vi "HEALTH_LABVIEW_V4.vi"() -> ()   [LabVIEW 2026]
uses:
  <vilib>/addons/control/pid/NI_PID_pid.lvlib
  <vilib>/addons/control/pid/pid.llb/PID (DBL).vi
panel:
  out "INTERMEDIATE BLOCK LOWER RTD":dbl format="%.2f"
  out "INTERMEDIATE BLOCK LOWER RTD":dbl(graph)
  out "OUTLET TEMP (C)":dbl
  out "INLET TEMP (C)":dbl
  out "INLET PRESSURE (PSI)":dbl format="%.2f"
  out "INLET PRESSURE (PSI)":dbl(graph)
  out "PRESSURE DROP (PSI)":dbl format="%.2f"
  out "PRESSURE DROP (PSI)":dbl(graph)
  out "DELTA T (C)":dbl
  in  "ZEROING DELTA T OFFSET":dbl
  out "DELTA T (C)":dbl(graph)
  out "COOLANT FLOW (LPM)":dbl(graph)
  out "COOLANT FLOW (LPM)":dbl
  in  "HTR PROP GAIN":dbl=3.0
  in  "PUMP SPEED CONTROL VOLTAGE":dbl(knob) scale=0.0..5.0
  in  "PUMP ON/OFF":bool
  out "HX TEMPERATURE (C)":dbl(graph)
  out "HEATER POWER OUTPUT":dbl(knob) scale=0.0..100.0
  in  "TARGET HX TEMP (C)":dbl
  in  "HEATER ON/OFF":bool
  out "HX TEMP (C)":dbl format="%.2f"
  in  "stop":bool
  out "Error String":string
  out "error out":errorcluster
  out "ConnectionType Out":i32
  out "DeviceType Out":i32
  in  "Identifier":string="LJM_idANY"
  in  "ConnectionType":string="LJM_ctANY"
  in  "DeviceType":string="LJM_dtANY"
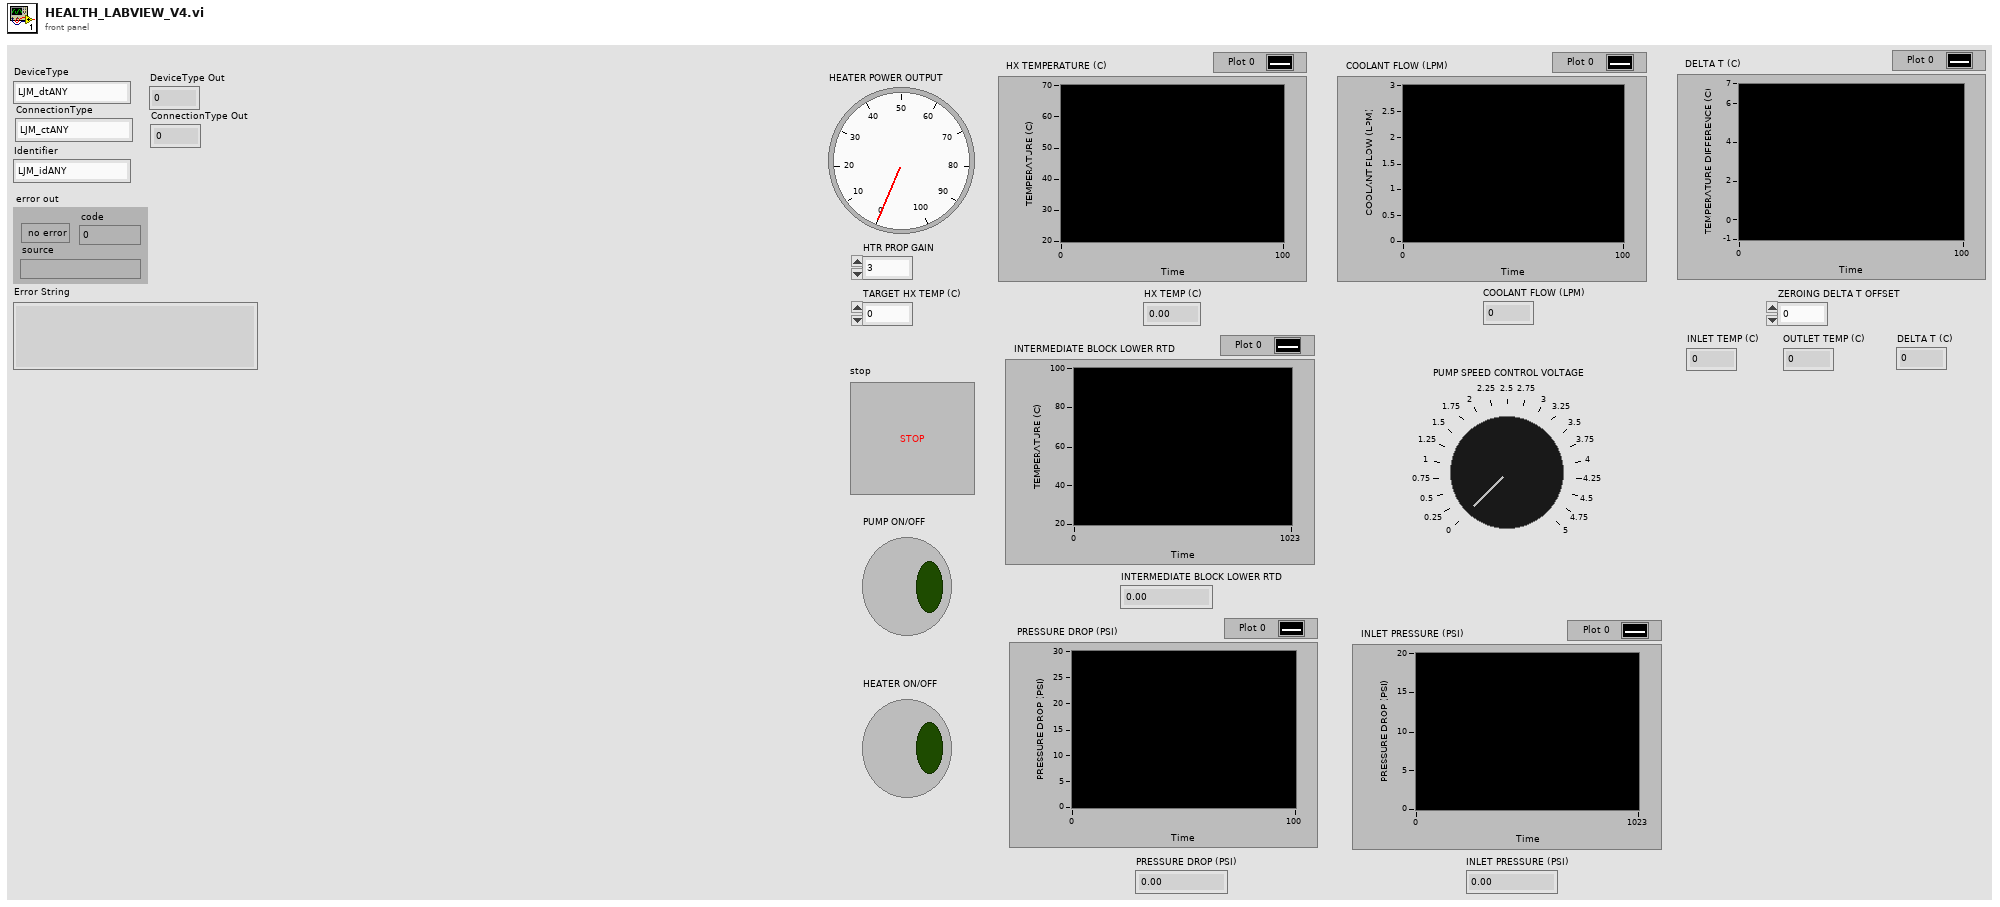
[diagram p1: front panel]
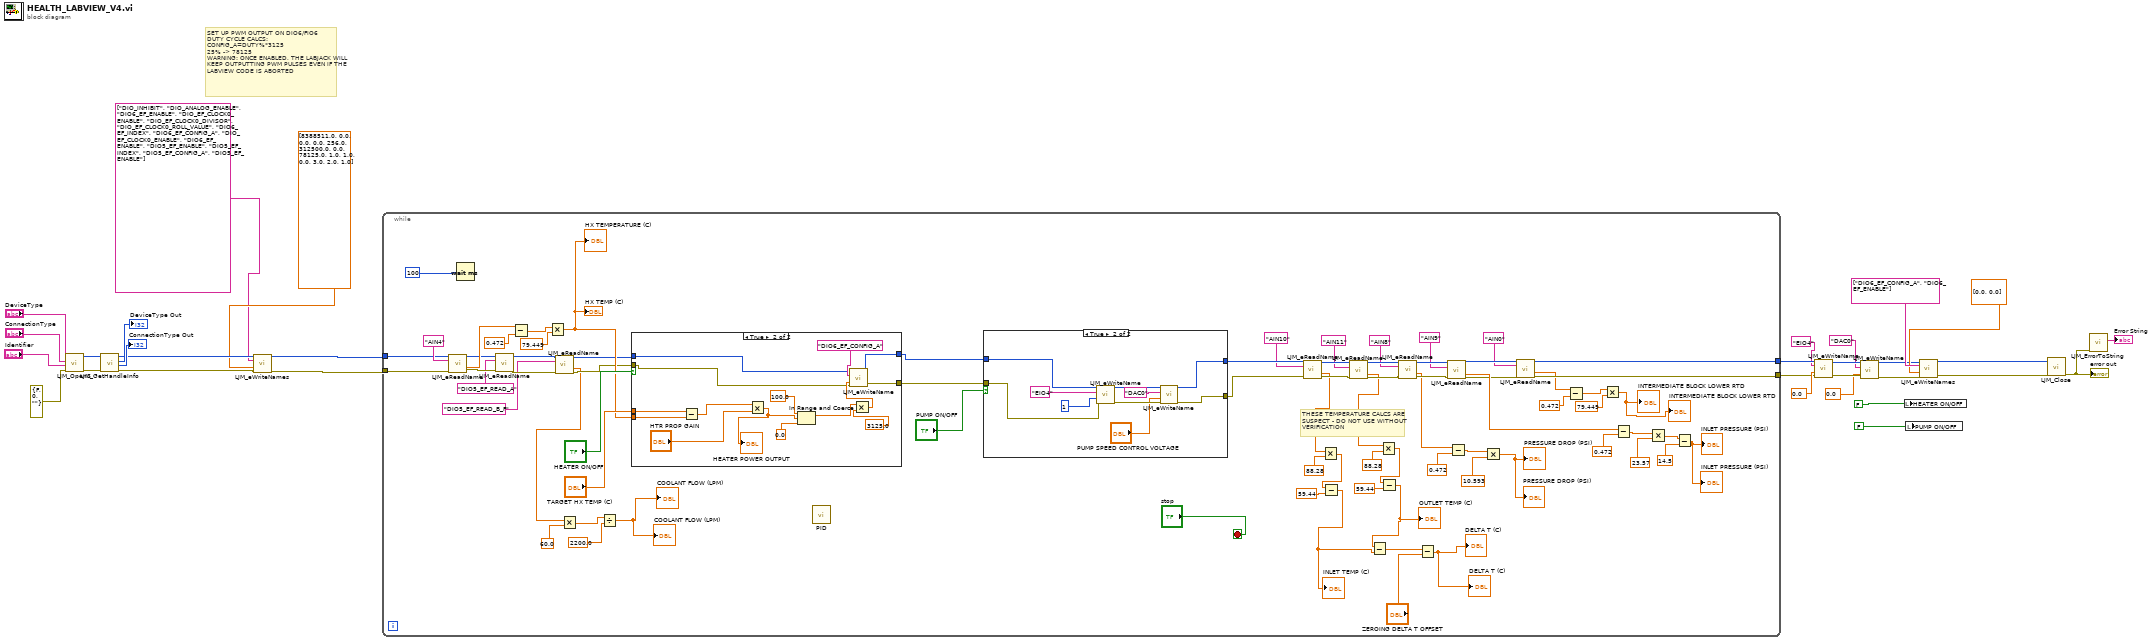
[diagram p0: block diagram]
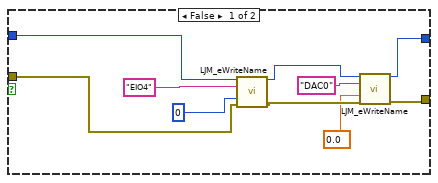
[diagram p2: hidden frame]
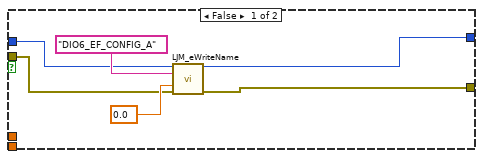
[diagram p3: hidden frame]
diagram:
  # "SET UP PWM OUTPUT ON DIO6/FIO6\nDUTY CYCLE CALCS:\nCONFIG_A=DUTY%*3125\n25% -> 78125\nWARNING: ONCE ENABLED, THE LABJACK WILL KEEP OUTPUTTING PWM PULSES EVEN IF THE LABVIEW CODE IS ABORTED"
  n1 = call "LJM_OpenS.vi"("error in"=errorcluster {"status"=FALSE, "code"=0, "source"=""} ("error in (no error)"), "Identifier"="Identifier", "ConnectionType"="ConnectionType", "DeviceType"="DeviceType") -> ("error out"=w31:errorcluster, "Handle"=w30:i32)  [unwired: 6 in]
  n2 = call "LJM_GetHandleInfo.vi"("error in"=w31, "Handle In"=w30) -> ("error out"=w21:errorcluster, "ConnectionType"=→"ConnectionType Out":i32, "DeviceType"=→"DeviceType Out":i32, "Handle Out"=w22:i32)  [unwired: 2 in, 4 out]
  n3 = call "LJM_eWriteNames.vi"("Handle In"=w22, "aNames"=string[] ["DIO_INHIBIT", "DIO_ANALOG_ENABLE", "DIO6_EF_ENABLE", "DIO_EF_CLOCK0_ENABLE", "DIO_EF_CLOCK0_DIVISOR", "DIO_EF_CLOCK0_ROLL_VALUE", "DIO6_EF_INDEX", "DIO6_EF_CONFIG_A", "DIO_EF_CLOCK0_ENABLE", "DIO6_EF_ENABLE", "DIO5_EF_ENABLE", "DIO5_EF_INDEX", "DIO5_EF_CONFIG_A", "DIO5_EF_ENABLE"], "aValuesIn"=dbl[] [8388511.0, 0.0, 0.0, 0.0, 256.0, 312500.0, 0.0, 78125.0, 1.0, 1.0, 0.0, 3.0, 2.0, 1.0], "error in"=w21) -> ("Handle Out"=w2:i32, "error out"=w1:errorcluster)  [unwired: 9 in, 1 out]
  n4 = while {
    tunnel: [w39] -> w9
    tunnel: w2 -> [w94]
    tunnel: w1 -> [w93]
    tunnel: [w40] -> w3
    stop <- "stop" stop-if-true
    # "THESE TEMPERATURE CALCS ARE SUSPECT - DO NOT USE WITHOUT VERIFICATION"
    n5 = call "LJM_eReadName.vi"("Handle In"=w94, "Name"="AIN4", "error in"=w93) -> ("Handle Out"=w92:i32, "Value"=w103:dbl, "error out"=w91:errorcluster)  [unwired: 10 in]
    n6 = Wait (ms)(milliseconds to wait=u32 100) -> ()  [unwired: 1 out]
    n7 = call "LJM_eReadName.vi"("Handle In"=w92, "Name"="DIO5_EF_READ_A", "error in"=w91) -> ("Handle Out"=w89:i32, "error out"=w86:errorcluster)  [unwired: 10 in, 1 out]
    n8 = Subtract(x=w103, y=0.472 ("Address 2")) -> (x-y=w106:dbl)
    n9 = Multiply(x=w106, y=79.449 ("Address 2")) -> (x*y=w98:dbl)
    "HX TEMP (C)" <- w98
    "HX TEMPERATURE (C)" <- w98
    n10 = call "LJM_eReadName.vi"("Handle In"=w89, "Name"="DIO5_EF_READ_B_F" ("DIO5_EF_READ_B_F"), "error in"=w86) -> ("Handle Out"=w88:i32, "Value"=w84:dbl, "error out"=w87:errorcluster)  [unwired: 10 in]
    n11 = Multiply(x=w84, y=60.0) -> (x*y=w82:dbl)
    n12 = Divide(x=w82, y=2200.0) -> (x/y=→"COOLANT FLOW (LPM)" →"COOLANT FLOW (LPM)":dbl)
    n13 = case shown="True" "HEATER ON/OFF" {
      tunnel: [w132 w148] -> w95
      tunnel: [w133 w147] -> w96
      tunnel: "TARGET HX TEMP (C)" -> [_ w143]
      tunnel: w98 -> [_ w142]
      tunnel: w88 -> [w129 w139]
      tunnel: w87 -> [w128 w138]
      frame False {
        n14 = call "LJM_eWriteName.vi"("Handle In"=w129, "Name"="DIO6_EF_CONFIG_A", "Value"=0.0, "error in"=w128) -> ("Handle Out"=w133:i32, "error out"=w132:errorcluster)  [unwired: 10 in]
      }
      frame True {
        n15 = Subtract(x=w143, y=w142) -> (x-y=w140:dbl)
        n16 = Multiply(x=w140, y="HTR PROP GAIN") -> (x*y=w137:dbl)
        "HEATER POWER OUTPUT" <- w137
        n17 = In Range and Coerce(upper limit=100.0, x=w137, lower limit=0.0) -> (coerced(x)=w134:dbl)  [unwired: 1 out]
        n18 = Multiply(x=w134, y=3125.0) -> (x*y=w145:dbl)
        n19 = call "LJM_eWriteName.vi"("Handle In"=w139, "Name"="DIO6_EF_CONFIG_A", "Value"=w145, "error in"=w138) -> ("Handle Out"=w147:i32, "error out"=w148:errorcluster)  [unwired: 10 in]
      }
    }
    n20 = call-poly <vilib>:"PID.vi"() -> ()  [unwired: 10 in, 2 out]
    n21 = case shown="True" "PUMP ON/OFF" {
      tunnel: w96 -> [w115 w125]
      tunnel: w95 -> [w114 w124]
      tunnel: [w110 w119] -> w75
      tunnel: [w109 w120] -> w79
      frame False {
        n22 = call "LJM_eWriteName.vi"("Handle In"=w115, "Name"="EIO4", "Value"=0, "error in"=w114) -> ("Handle Out"=w112:i32, "error out"=w111:errorcluster)  [unwired: 10 in]
        n23 = call "LJM_eWriteName.vi"("Handle In"=w112, "Name"="DAC0", "Value"=0.0, "error in"=w111) -> ("Handle Out"=w109:i32, "error out"=w110:errorcluster)  [unwired: 10 in]
      }
      frame True {
        n24 = call "LJM_eWriteName.vi"("Handle In"=w125, "Name"="EIO4", "Value"=1, "error in"=w124) -> ("Handle Out"=w121:i32, "error out"=w122:errorcluster)  [unwired: 10 in]
        n25 = call "LJM_eWriteName.vi"("Handle In"=w121, "Name"="DAC0", "Value"="PUMP SPEED CONTROL VOLTAGE", "error in"=w122) -> ("Handle Out"=w120:i32, "error out"=w119:errorcluster)  [unwired: 10 in]
      }
    }
    n26 = call "LJM_eReadName.vi"("Handle In"=w79, "Name"="AIN10", "error in"=w75) -> ("Handle Out"=w78:i32, "Value"=w67:dbl, "error out"=w74:errorcluster)  [unwired: 10 in]
    n27 = Multiply(x=w67, y=88.28) -> (x*y=w65:dbl)
    n28 = Subtract(x=w65, y=59.44) -> (x-y=w45:dbl)
    "INLET TEMP (C)" <- w45
    n29 = call "LJM_eReadName.vi"("Handle In"=w78, "Name"="AIN11" ("Name 2"), "error in"=w74) -> ("Handle Out"=w77:i32, "Value"=w60:dbl, "error out"=w73:errorcluster)  [unwired: 10 in]
    n30 = Multiply(x=w60, y=88.28) -> (x*y=w62:dbl)
    n31 = Subtract(x=w62, y=59.44) -> (x-y=w44:dbl)
    "OUTLET TEMP (C)" <- w44
    n32 = Subtract(x=w44, y=w45) -> (x-y=w59:dbl)
    n33 = call "LJM_eReadName.vi"("Handle In"=w77, "Name"="AIN8" ("Name 3"), "error in"=w73) -> ("Handle Out"=w76:i32, "Value"=w43:dbl, "error out"=w72:errorcluster)  [unwired: 10 in]
    n34 = Subtract(x=w59, y="ZEROING DELTA T OFFSET") -> (x-y=→"DELTA T (C)" →"DELTA T (C)":dbl)
    n35 = call "LJM_eReadName.vi"("Handle In"=w76, "Name"="AIN9" ("Name 4"), "error in"=w72) -> ("Handle Out"=w42:i32, "Value"=w49:dbl, "error out"=w41:errorcluster)  [unwired: 10 in]
    n36 = Subtract(x=w43, y=0.472) -> (x-y=w55:dbl)
    n37 = Multiply(x=w55, y=10.593) -> (x*y=→"PRESSURE DROP (PSI)" →"PRESSURE DROP (PSI)":dbl)
    n38 = call "LJM_eReadName.vi"("Handle In"=w42, "Name"="AIN0", "error in"=w41) -> ("Handle Out"=w39:i32, "Value"=w34:dbl, "error out"=w40:errorcluster)  [unwired: 10 in]
    n39 = Subtract(x=w34, y=0.472 ("Address 2")) -> (x-y=w37:dbl)
    n40 = Multiply(x=w37, y=79.449 ("Address 2")) -> (x*y=→"INTERMEDIATE BLOCK LOWER RTD" →"INTERMEDIATE BLOCK LOWER RTD":dbl)
    n41 = Subtract(x=w49, y=0.472) -> (x-y=w51:dbl)
    n42 = Multiply(x=w51, y=23.57) -> (x*y=w47:dbl)
    n43 = Subtract(x=w47, y=14.5) -> (x-y=→"INLET PRESSURE (PSI)" →"INLET PRESSURE (PSI)":dbl)
  }
  n44 = call "LJM_eWriteName.vi"("Handle In"=w9, "Name"="EIO4", "Value"=0.0, "error in"=w3) -> ("Handle Out"=w10:i32, "error out"=w13:errorcluster)  [unwired: 10 in]
  n45 = call "LJM_eWriteName.vi"("Handle In"=w10, "Name"="DAC0", "Value"=0.0, "error in"=w13) -> ("Handle Out"=w11:i32, "error out"=w12:errorcluster)  [unwired: 10 in]
  n46 = local write "HEATER ON/OFF"(FALSE ("HEATER ON/OFF 2")) -> ()
  n47 = local write "PUMP ON/OFF"(FALSE ("PUMP ON/OFF 2")) -> ()
  n48 = call "LJM_eWriteNames.vi"("Handle In"=w11, "aNames"=string[] ["DIO6_EF_CONFIG_A", "DIO6_EF_ENABLE"], "aValuesIn"=dbl[] [0.0, 0.0], "error in"=w12) -> ("Handle Out"=w17:i32, "error out"=w18:errorcluster)  [unwired: 9 in, 1 out]
  n49 = call "LJM_Close.vi"("error in"=w18, "Handle"=w17) -> ("error out"=w23:errorcluster)  [unwired: 9 in]
  "error out" <- w23
  n50 = call "LJM_ErrorToString.vi"("error in"=w23) -> ("String"=→"Error String":string)  [unwired: 10 in]
